vi "test_libssh2_crypto_engine.vi"() -> ()   [LabVIEW 2017, in "unit_tests.lvlib"]
uses:
  unit_tests.lvlib
  libssh2/libssh2_crypto_engine.ctl
  libssh2/libssh2_init_default.vi
  libssh2/libssh2.lvlib
  <vilib>/PNR/Transparent Assertions/Transparent Assertions/Transparent Assertions.lvlib
panel:
  out "error out":errorcluster
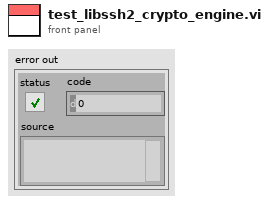
[diagram p1: front panel]
types:
  T1 = typedef "libssh2.lvlib/libssh2_crypto_engine.ctl" = enum16{"no crypto", "OpenSSL", "gcrypt", "mbedTLS", "WinCNG", "OS400qc3"}
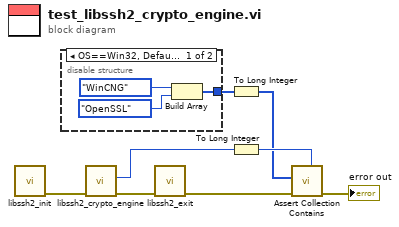
[diagram p0: block diagram]
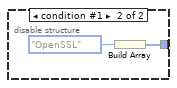
[diagram p2: hidden frame]
diagram:
  n1 = call-poly "libssh2_init.vi"() -> ("error out"=w8:errorcluster)  [unwired: 11 in]
  n2 = disable-structure shown="OS==Win32, Default" {
    disable-tunnel: [w10 w12] -> w4
    frame condition #0 (active) {
      n3 = Build Array(libssh2_crypto_engine."WinCNG" ("crypto engine"), libssh2_crypto_engine."OpenSSL" ("crypto engine")) -> (w10:T1[])
    }
    frame condition #1 {
      n4 = Build Array(libssh2_crypto_engine."OpenSSL" ("crypto engine")) -> (w12:T1[])
    }
  }
  n5 = call "libssh2_crypto_engine.vi"("error in (no error)"=w8) -> ("error out"=w6:errorcluster, "crypto engine"=w3:T1)  [unwired: 9 in]
  n6 = call "libssh2_exit.vi"("error in (no error)"=w6) -> ("error out"=w7:errorcluster)  [unwired: 10 in]
  n7 = To Long Integer(number=w4) -> (32bit integer=w1:i32[])
  n8 = To Long Integer(number=w3) -> (32bit integer=w2:i32)
  n9 = call <vilib>:"Assert Collection Contains.vi"("Expected"=w2, "error in (no error)"=w7, "Collection"=w1) -> ("error out"=→"error out":errorcluster)  [unwired: 8 in]
